vi "Do Request.vi"(8 "error in (no error)":errorcluster, 10 "request.lvclass":refnum<class "request.lvclass">, 11 "output_actor in":refnum<class "Output Actor.lvclass">) -> (0 "error out":errorcluster, 3 "output_actor out":refnum<class "Output Actor.lvclass">)   [LabVIEW 2015, in "Output Actor.lvclass"]
uses:
  Output Actor.lvclass
  Request/request.lvclass
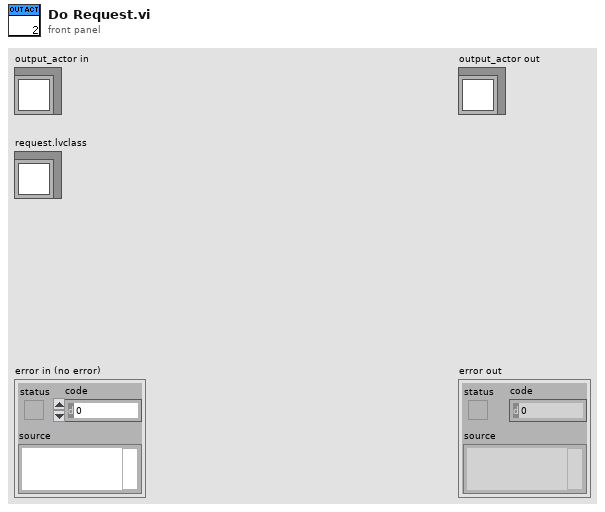
[diagram p1: front panel]
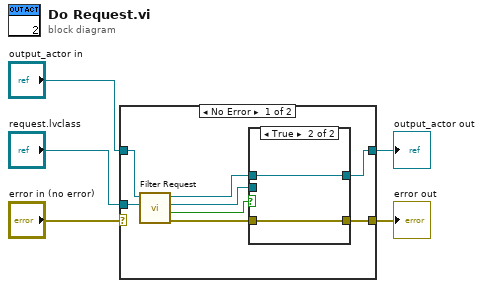
[diagram p0: block diagram]
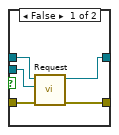
[diagram p2: hidden frame]
diagram:
  n1 = case shown="No Error" "error in (no error)" {
    selector: "error in (no error)" -> [_ w22]
    tunnel: [w12 w22] -> w4
    tunnel: [w13 w21] -> w2
    tunnel: "output_actor in" -> [w11 w21]
    tunnel: "request.lvclass" -> [w10 _]
    frame No Error {
      n2 = call-dynamic "Filter Request.vi"("request"=w10, "output_actor in"=w11) -> ("error out"=w7:errorcluster, "Filtered"=w6:bool, "request out"=w9:refnum<class "request.lvclass">, "output_actor out"=w8:refnum<class "Output Actor.lvclass">)  [unwired: 6 in]
      n3 = case shown="True" w6 {
        tunnel: [w18 w20] -> w13
        tunnel: [w17 w19] -> w12
        tunnel: w9 -> [w16 _]
        tunnel: w8 -> [w15 w20]
        tunnel: w7 -> [w14 w19]
        frame False {
          n4 = call-dynamic "Request.vi"("error in (no error)"=w14, "request"=w16, "output_actor in"=w15) -> ("error out"=w17:errorcluster, "output_actor out"=w18:refnum<class "Output Actor.lvclass">)  [unwired: 7 in]
        }
        frame True {
        }
      }
    }
    frame Error {
    }
  }
  "error out" <- w4
  "output_actor out" <- w2
